vi "Initialize DAQ.vi"(0 "number of samples":i32=100, 1 "rate":dbl=1000.0, 2 "System Type":T1, 3 "System Ref":tag) -> (14 "AI Task OUT":refnum<k21> caption="Input Task OUT", 15 "Ctr Present":bool, 16 "Ctr Task OUT":refnum<k21>, 19 "error out":errorcluster)   [LabVIEW 2023]
uses:
  Type Defs and Controls/System Type.ctl
  <vilib>/DAQmx/read.llb/DAQmx Read (Analog 2D DBL NChan NSamp).vi
  <vilib>/DAQmx/create/channels.llb/DAQmx Create Channel (AI-Voltage-Basic).vi
  <vilib>/DAQmx/create/channels.llb/DAQmx Create Channel (AI-Current-Basic).vi
  <vilib>/DAQmx/create/channels.llb/DAQmx Create Channel (AI-Temperature-Thermocouple).vi
  <vilib>/DAQmx/create/channels.llb/DAQmx Create Channel (CI-Count Edges).vi
  <vilib>/DAQmx/configure/timing.llb/DAQmx Timing (Sample Clock).vi
  <vilib>/DAQmx/miscellaneous.llb/DAQmx Fill In Error Info.vi
  <resource>/objmgr/daqmx.rc
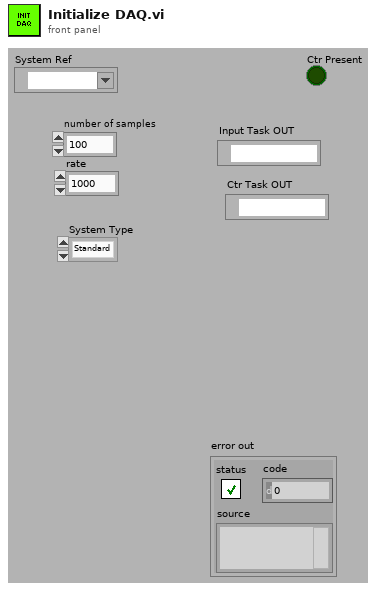
[diagram p1: front panel]
types:
  T1 = typedef "System Type.ctl" = enum16{"Standard", "Deformation", "Standard 8TC"}
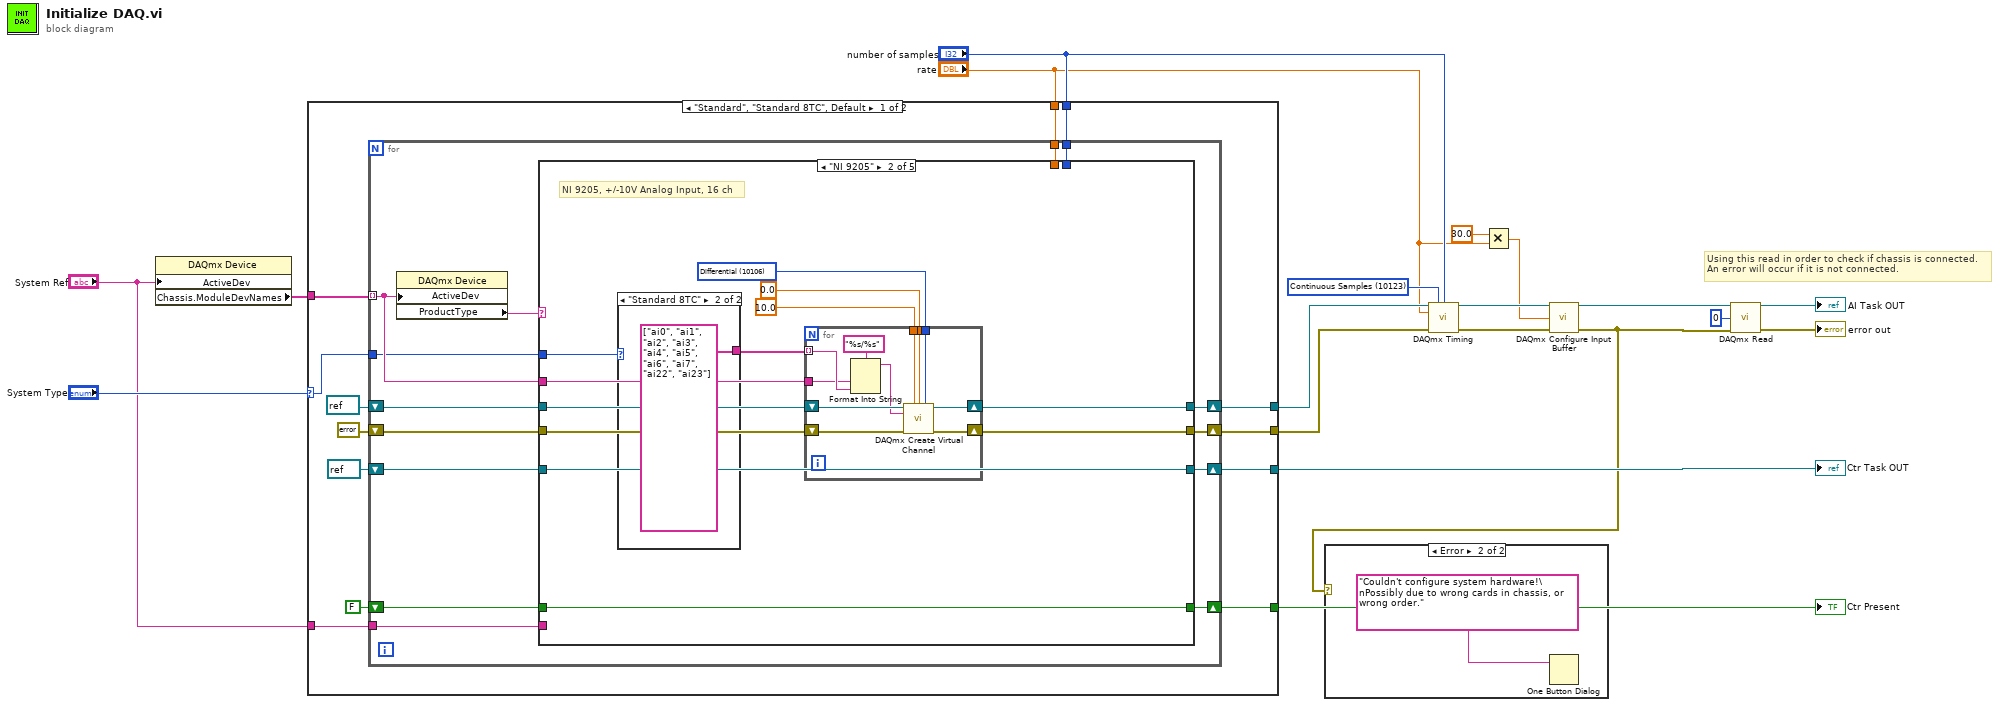
[diagram p0: block diagram]
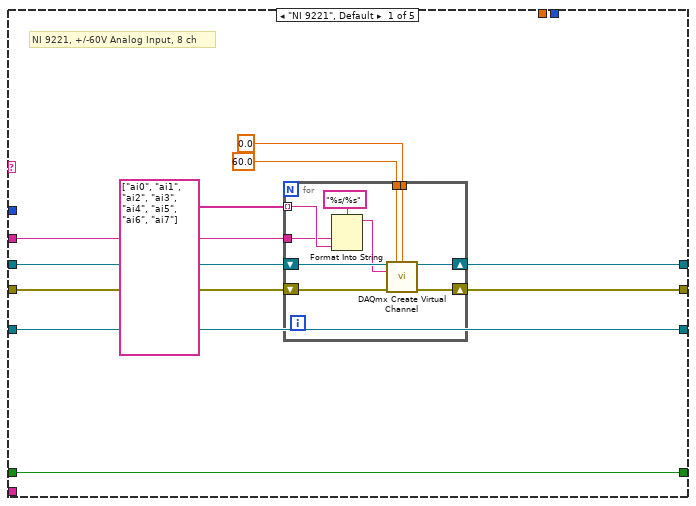
[diagram p2: hidden frame]
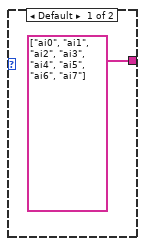
[diagram p3: hidden frame]
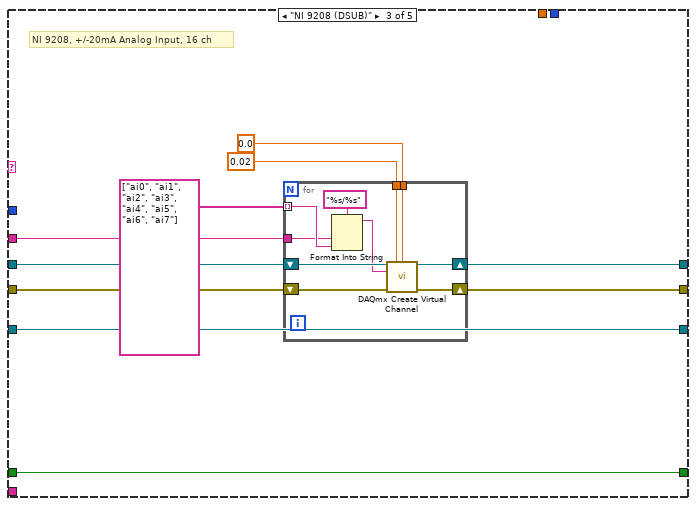
[diagram p4: hidden frame]
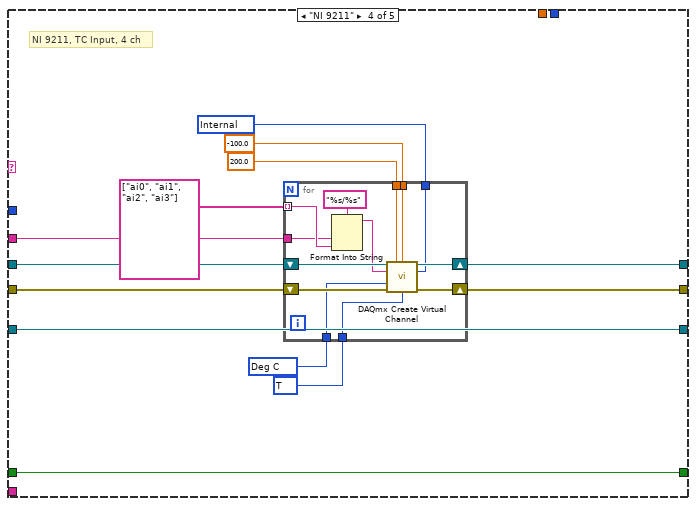
[diagram p5: hidden frame]
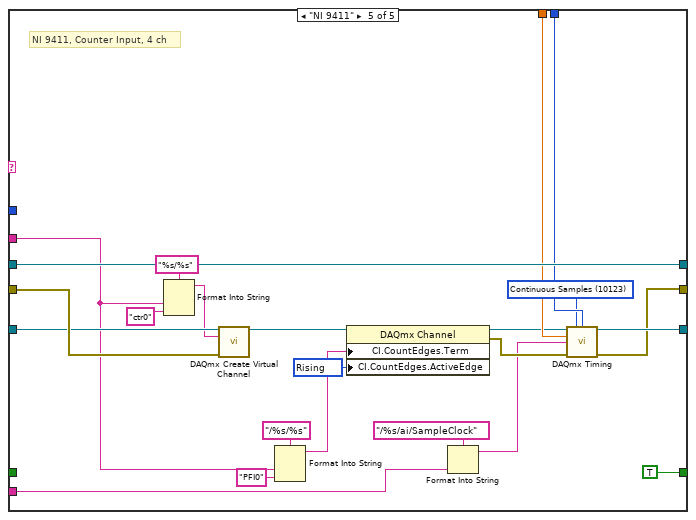
[diagram p6: hidden frame]
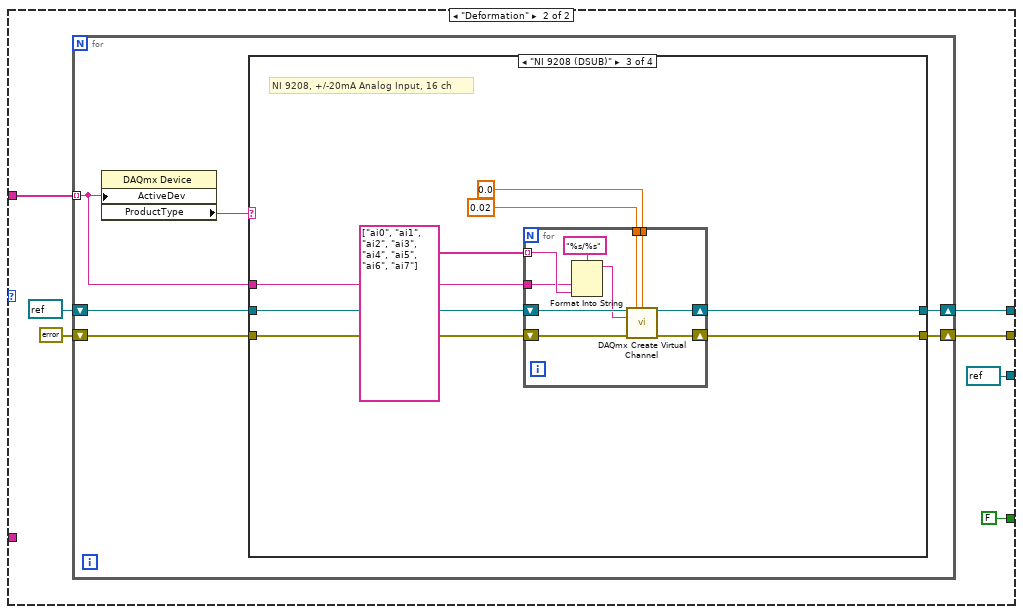
[diagram p7: hidden frame]
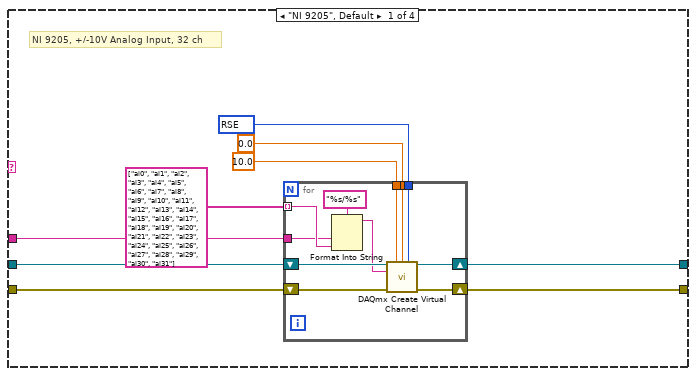
[diagram p8: hidden frame]
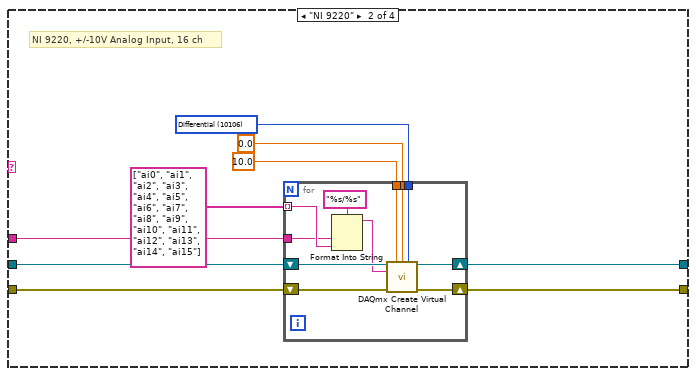
[diagram p9: hidden frame]
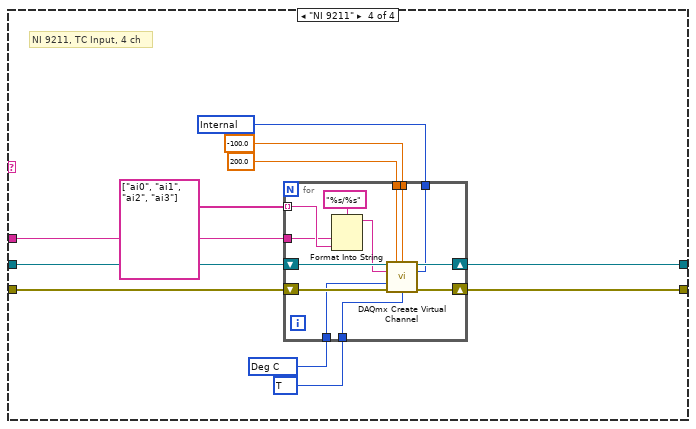
[diagram p10: hidden frame]
diagram:
  w10 = 10123 items=["Finite Samples"=10178, "Continuous Samples"=10123, "Hardware Timed Single Point"=12522] ("sample mode")
  # "Using this read in order to check if chassis is connected.\nAn error will occur if it is not connected."
  n1 = property class="DAQmx Device"("ActiveDev"="System Ref") -> ("Chassis.ModuleDevNames"=w9:tag[])  [unwired: 2 in, 2 out]
  n2 = case shown="\"Standard\", \"Standard 8TC\", Default" "System Type" {
    selector: "System Type" -> [w20 _]
    tunnel: w9 -> [w32 w167]
    tunnel: [w29 w164] -> w12
    tunnel: [w28 w163] -> w11
    tunnel: [w27 FALSE] -> w16
    tunnel: [w24 refnum<k21> refnum ("task out")] -> w15
    tunnel: "rate" -> [w23 _]
    tunnel: "number of samples" -> [w22 _]
    tunnel: "System Ref" -> [w21 _]
    frame "Standard", "Standard 8TC", Default {
      n3 = for {
        tunnel: w32 -> [w45] mode=indexing
        shift-right: [w42] -> w29
        shift-left: refnum<k21> refnum ("task out") -> [w44]
        shift-right: [w41] -> w28
        shift-left: errorcluster {"status"=FALSE, "code"=0, "source"=""} ("error out") -> [w43]
        shift-right: [w40] -> w27
        shift-left: FALSE -> [w39]
        shift-right: [w38] -> w24
        shift-left: refnum<k21> refnum ("task out") -> [w37]
        tunnel: w23 -> [w36]
        tunnel: w22 -> [w35]
        tunnel: w21 -> [w34]
        tunnel: w20 -> [w33]
        n4 = property class="DAQmx Device"("ActiveDev"=w45) -> ("ProductType"=w46:string)  [unwired: 2 in, 2 out]
        n5 = case shown="\"NI 9205\"" w46 {
          tunnel: w45 -> [w53 w75 w98 w121 w150]
          tunnel: w44 -> [w52 w74 w97 w120 w157]
          tunnel: w43 -> [w51 w73 w96 w119 w160]
          tunnel: [w50 w72 w95 w118 w157] -> w42
          tunnel: [w49 w71 w94 w117 w152] -> w41
          tunnel: [w48 w69 w93 w113 TRUE] -> w40
          tunnel: w39 -> [w48 w69 w93 w113 _]
          tunnel: [w47 w68 w92 w112 w153] -> w38
          tunnel: w37 -> [w47 w68 w92 w112 w158]
          tunnel: w36 -> [_ _ _ _ w156]
          tunnel: w35 -> [_ _ _ _ w155]
          tunnel: w34 -> [_ _ _ _ w140]
          tunnel: w33 -> [_ w67 _ _ _]
          frame "NI 9221", Default {
            # "NI 9221, +/-60V Analog Input, 8 ch"
            n6 = for {
              tunnel: 0.0 ("minimum value") -> [w65]
              tunnel: 60.0 ("maximum value") -> [w66]
              tunnel: string[] ["ai0", "ai1", "ai2", "ai3", "ai4", "ai5", "ai6", "ai7"] ("Array") -> [w61] mode=indexing
              shift-right: [w58] -> w49
              shift-left: w51 -> [w63]
              shift-right: [w62] -> w50
              shift-left: w52 -> [w64]
              tunnel: w53 -> [w57]
              n7 = Format Into String(format string="%s/%s", w57, w61) -> (resulting string=w59:string)  [unwired: 2 in, 1 out]
              n8 = call-poly <vilib>:"DAQmx Create Virtual Channel.vi"("task in"=w64, "maximum value"=w66, "minimum value"=w65, "physical channels"=w59, "error in"=w63) -> ("task out"=w62:refnum<k21>, "error out"=w58:errorcluster)  [unwired: 9 in]
            }
          }
          frame "NI 9205" {
            w70 = 10106 items=["default"=-1, "RSE"=10083, "NRSE"=10078, "Differential"=10106, "Pseudodifferential"=12529] ("input terminal configuration")
            # "NI 9205, +/-10V Analog Input, 16 ch"
            n9 = case shown="\"Standard 8TC\"" w67 {
              tunnel: [string[] ["ai0", "ai1", "ai2", "ai3", "ai4", "ai5", "ai6", "ai7"] ("Array") string[] ["ai0", "ai1", "ai2", "ai3", "ai4", "ai5", "ai6", "ai7", "ai22", "ai23"] ("Array")] -> w76
              frame Default {
              }
              frame "Standard 8TC" {
              }
            }
            n10 = for {
              tunnel: 0.0 ("minimum value") -> [w90]
              tunnel: 10.0 ("maximum value") -> [w91]
              tunnel: w76 -> [w86] mode=indexing
              shift-right: [w83] -> w71
              shift-left: w73 -> [w88]
              shift-right: [w87] -> w72
              shift-left: w74 -> [w89]
              tunnel: w75 -> [w82]
              tunnel: w70 -> [w81]
              n11 = Format Into String(format string="%s/%s", w82, w86) -> (resulting string=w84:string)  [unwired: 2 in, 1 out]
              n12 = call-poly <vilib>:"DAQmx Create Virtual Channel.vi"("task in"=w89, "maximum value"=w91, "minimum value"=w90, "input terminal configuration"=w81, "physical channels"=w84, "error in"=w88) -> ("task out"=w87:refnum<k21>, "error out"=w83:errorcluster)  [unwired: 8 in]
            }
          }
          frame "NI 9208 (DSUB)" {
            # "NI 9208, +/-20mA Analog Input, 16 ch"
            n13 = for {
              tunnel: 0.0 ("minimum value") -> [w110]
              tunnel: 0.02 ("maximum value") -> [w111]
              tunnel: string[] ["ai0", "ai1", "ai2", "ai3", "ai4", "ai5", "ai6", "ai7"] ("Array") -> [w106] mode=indexing
              shift-right: [w103] -> w94
              shift-left: w96 -> [w108]
              shift-right: [w107] -> w95
              shift-left: w97 -> [w109]
              tunnel: w98 -> [w102]
              n14 = Format Into String(format string="%s/%s", w102, w106) -> (resulting string=w104:string)  [unwired: 2 in, 1 out]
              n15 = call-poly <vilib>:"DAQmx Create Virtual Channel.vi"("task in"=w109, "maximum value"=w111, "minimum value"=w110, "physical channels"=w104, "error in"=w108) -> ("task out"=w107:refnum<k21>, "error out"=w103:errorcluster)  [unwired: 9 in]
            }
          }
          frame "NI 9211" {
            w114 = 10086 items=["J"=10072, "K"=10073, "N"=10077, "R"=10082, "S"=10085, "T"=10086, "B"=10047, "E"=10055] ("thermocouple type")
            w115 = 10143 items=["Deg C"=10143, "Deg F"=10144, "Kelvins"=10325, "Deg R"=10145, "From Custom Scale"=10065] ("units")
            w116 = u32 10200 items=["Internal"=10200, "Constant Value"=10116, "Channel"=10113] ("cjc source")
            # "NI 9211, TC Input, 4 ch"
            n16 = for {
              tunnel: -100.0 ("minimum value") -> [w136]
              tunnel: 200.0 ("maximum value") -> [w137]
              tunnel: string[] ["ai0", "ai1", "ai2", "ai3"] ("Array") -> [w132] mode=indexing
              shift-right: [w129] -> w117
              shift-left: w119 -> [w134]
              shift-right: [w133] -> w118
              shift-left: w120 -> [w135]
              tunnel: w121 -> [w128]
              tunnel: w116 -> [w127]
              tunnel: w115 -> [w126]
              tunnel: w114 -> [w125]
              n17 = Format Into String(format string="%s/%s", w128, w132) -> (resulting string=w130:string)  [unwired: 2 in, 1 out]
              n18 = call-poly <vilib>:"DAQmx Create Virtual Channel.vi"("task in"=w135, "maximum value"=w137, "minimum value"=w136, "physical channels"=w130, "cjc source"=w127, "units"=w126, "error in"=w134, "thermocouple type"=w125) -> ("task out"=w133:refnum<k21>, "error out"=w129:errorcluster)  [unwired: 6 in]
            }
          }
          frame "NI 9411" {
            w143 = 10280 items=["Rising"=10280, "Falling"=10171] ("CI.CountEdges.ActiveEdge")
            w154 = 10123 items=["Finite Samples"=10178, "Continuous Samples"=10123, "Hardware Timed Single Point"=12522] ("sample mode")
            # "NI 9411, Counter Input, 4 ch"
            n19 = Format Into String(format string="%s/%s", w150, "ctr0" ("physical channel")) -> (resulting string=w147:string)  [unwired: 2 in, 1 out]
            n20 = call-poly <vilib>:"DAQmx Create Virtual Channel.vi"("task in"=w158, "counter"=w147, "error in"=w160) -> ("task out"=w145:refnum<k21>)  [unwired: 11 in, 1 out]
            n21 = Format Into String(format string="/%s/%s", w150, "PFI0" ("input 2")) -> (resulting string=w144:string)  [unwired: 2 in, 1 out]
            n22 = property class="DAQmx Channel"(reference=w145, "CI.CountEdges.Term"=w144, "CI.CountEdges.ActiveEdge"=w143) -> (reference out=w142:refnum<k21>, error out=w141:errorcluster)  [unwired: 1 in]
            n23 = Format Into String(format string="/%s/ai/SampleClock", w140) -> (resulting string=w138:string)  [unwired: 2 in, 1 out]
            n24 = call-poly <vilib>:"DAQmx Timing.vi"("task/channels in"=w142, "sample mode"=w154, "samples per channel"=w155, "rate"=w156, "source"=w138, "error in"=w141) -> ("task out"=w153:refnum<k21>, "error out"=w152:errorcluster)  [unwired: 8 in]
          }
        }
      }
    }
    frame "Deformation" {
      n25 = for {
        tunnel: w167 -> [w172] mode=indexing
        shift-right: [w169] -> w164
        shift-left: refnum<k21> refnum ("task out") -> [w171]
        shift-right: [w168] -> w163
        shift-left: errorcluster {"status"=FALSE, "code"=0, "source"=""} ("error out") -> [w170]
        n26 = property class="DAQmx Device"("ActiveDev"=w172) -> ("ProductType"=w173:string)  [unwired: 2 in, 2 out]
        n27 = case shown="\"NI 9208 (DSUB)\"" w173 {
          tunnel: w172 -> [w180 w200 w218 w239]
          tunnel: w171 -> [w179 w199 w217 w238]
          tunnel: w170 -> [w178 w198 w216 w237]
          tunnel: [w177 w197 w215 w236] -> w169
          tunnel: [w176 w196 w214 w235] -> w168
          frame "NI 9205", Default {
            w175 = 10083 items=["default"=-1, "RSE"=10083, "NRSE"=10078, "Differential"=10106, "Pseudodifferential"=12529] ("input terminal configuration")
            # "NI 9205, +/-10V Analog Input, 32 ch"
            n28 = for {
              tunnel: 0.0 ("minimum value") -> [w192]
              tunnel: 10.0 ("maximum value") -> [w193]
              tunnel: string[] ["ai0", "ai1", "ai2", "ai3", "ai4", "ai5", "ai6", "ai7", "ai8", "ai9", "ai10", "ai11", "ai12", "ai13", "ai14", "ai15", "ai16", "ai17", "ai18", "ai19", "ai20", "ai21", "ai22", "ai23", "ai24", "ai25", "ai26", "ai27", "ai28", "ai29", "ai30", "ai31"] ("Array") -> [w188] mode=indexing
              shift-right: [w185] -> w176
              shift-left: w178 -> [w190]
              shift-right: [w189] -> w177
              shift-left: w179 -> [w191]
              tunnel: w180 -> [w184]
              tunnel: w175 -> [w183]
              n29 = Format Into String(format string="%s/%s", w184, w188) -> (resulting string=w186:string)  [unwired: 2 in, 1 out]
              n30 = call-poly <vilib>:"DAQmx Create Virtual Channel.vi"("task in"=w191, "maximum value"=w193, "minimum value"=w192, "input terminal configuration"=w183, "physical channels"=w186, "error in"=w190) -> ("task out"=w189:refnum<k21>, "error out"=w185:errorcluster)  [unwired: 8 in]
            }
          }
          frame "NI 9220" {
            w195 = 10106 items=["default"=-1, "RSE"=10083, "NRSE"=10078, "Differential"=10106, "Pseudodifferential"=12529] ("input terminal configuration")
            # "NI 9220, +/-10V Analog Input, 16 ch"
            n31 = for {
              tunnel: 0.0 ("minimum value") -> [w212]
              tunnel: 10.0 ("maximum value") -> [w213]
              tunnel: string[] ["ai0", "ai1", "ai2", "ai3", "ai4", "ai5", "ai6", "ai7", "ai8", "ai9", "ai10", "ai11", "ai12", "ai13", "ai14", "ai15"] ("Array") -> [w208] mode=indexing
              shift-right: [w205] -> w196
              shift-left: w198 -> [w210]
              shift-right: [w209] -> w197
              shift-left: w199 -> [w211]
              tunnel: w200 -> [w204]
              tunnel: w195 -> [w203]
              n32 = Format Into String(format string="%s/%s", w204, w208) -> (resulting string=w206:string)  [unwired: 2 in, 1 out]
              n33 = call-poly <vilib>:"DAQmx Create Virtual Channel.vi"("task in"=w211, "maximum value"=w213, "minimum value"=w212, "input terminal configuration"=w203, "physical channels"=w206, "error in"=w210) -> ("task out"=w209:refnum<k21>, "error out"=w205:errorcluster)  [unwired: 8 in]
            }
          }
          frame "NI 9208 (DSUB)" {
            # "NI 9208, +/-20mA Analog Input, 16 ch"
            n34 = for {
              tunnel: 0.0 ("minimum value") -> [w230]
              tunnel: 0.02 ("maximum value") -> [w231]
              tunnel: string[] ["ai0", "ai1", "ai2", "ai3", "ai4", "ai5", "ai6", "ai7"] ("Array") -> [w226] mode=indexing
              shift-right: [w223] -> w214
              shift-left: w216 -> [w228]
              shift-right: [w227] -> w215
              shift-left: w217 -> [w229]
              tunnel: w218 -> [w222]
              n35 = Format Into String(format string="%s/%s", w222, w226) -> (resulting string=w224:string)  [unwired: 2 in, 1 out]
              n36 = call-poly <vilib>:"DAQmx Create Virtual Channel.vi"("task in"=w229, "maximum value"=w231, "minimum value"=w230, "physical channels"=w224, "error in"=w228) -> ("task out"=w227:refnum<k21>, "error out"=w223:errorcluster)  [unwired: 9 in]
            }
          }
          frame "NI 9211" {
            w232 = 10086 items=["J"=10072, "K"=10073, "N"=10077, "R"=10082, "S"=10085, "T"=10086, "B"=10047, "E"=10055] ("thermocouple type")
            w233 = 10143 items=["Deg C"=10143, "Deg F"=10144, "Kelvins"=10325, "Deg R"=10145, "From Custom Scale"=10065] ("units")
            w234 = u32 10200 items=["Internal"=10200, "Constant Value"=10116, "Channel"=10113] ("cjc source")
            # "NI 9211, TC Input, 4 ch"
            n37 = for {
              tunnel: -100.0 ("minimum value") -> [w254]
              tunnel: 200.0 ("maximum value") -> [w255]
              tunnel: string[] ["ai0", "ai1", "ai2", "ai3"] ("Array") -> [w250] mode=indexing
              shift-right: [w247] -> w235
              shift-left: w237 -> [w252]
              shift-right: [w251] -> w236
              shift-left: w238 -> [w253]
              tunnel: w239 -> [w246]
              tunnel: w234 -> [w245]
              tunnel: w233 -> [w244]
              tunnel: w232 -> [w243]
              n38 = Format Into String(format string="%s/%s", w246, w250) -> (resulting string=w248:string)  [unwired: 2 in, 1 out]
              n39 = call-poly <vilib>:"DAQmx Create Virtual Channel.vi"("task in"=w253, "maximum value"=w255, "minimum value"=w254, "physical channels"=w248, "cjc source"=w245, "units"=w244, "error in"=w252, "thermocouple type"=w243) -> ("task out"=w251:refnum<k21>, "error out"=w247:errorcluster)  [unwired: 6 in]
            }
          }
        }
      }
    }
  }
  "Ctr Present" <- w16
  "Ctr Task OUT" <- w15
  n40 = call-poly <vilib>:"DAQmx Timing.vi"("task/channels in"=w12, "sample mode"=w10, "samples per channel"="number of samples", "rate"="rate", "error in"=w11) -> ("task out"=w8:refnum<k21>, "error out"=w6:errorcluster)  [unwired: 9 in]
  n41 = Multiply(x=30.0, y="rate") -> (x*y=w2:dbl)
  n42 = call <vilib>:"DAQmx Configure Input Buffer.vi"("task/channels in"=w8, "buffer size (in samples per channel)"=w2, "error in"=w6) -> ("task out"=w7:refnum<k21>, "error out"=w5:errorcluster)  [unwired: 11 in]
  n43 = case shown="Error" w5 {
    frame No Error {
    }
    frame Error {
      n44 = One Button Dialog(message="Couldn't configure system hardware!\nPossibly due to wrong cards in chassis, or wrong order.") -> ()  [unwired: 1 in, 1 out]
    }
  }
  n45 = call-poly <vilib>:"DAQmx Read.vi"("task/channels in"=w7, "number of samples per channel"=0, "error in"=w5) -> ("task out"=→"AI Task OUT":refnum<k21>, "error out"=→"error out":errorcluster)  [unwired: 10 in, 1 out]
